vi "Deposit Amount.vi"(10 "User Input":string, 11 "Module Data in":T1) -> (2 "Deposit Complete Message":string, 3 "Module Data out":T1)   [LabVIEW 2016]
uses:
  <vilib>/Utility/file.llb/Write Delimited Spreadsheet (string).vi
  Controls/UI Controls.ctl
  Controls/ATM Messages.ctl
  Controls/Transaction Status.ctl
  Controls/User Input Data.ctl
  Controls/Module Data.ctl
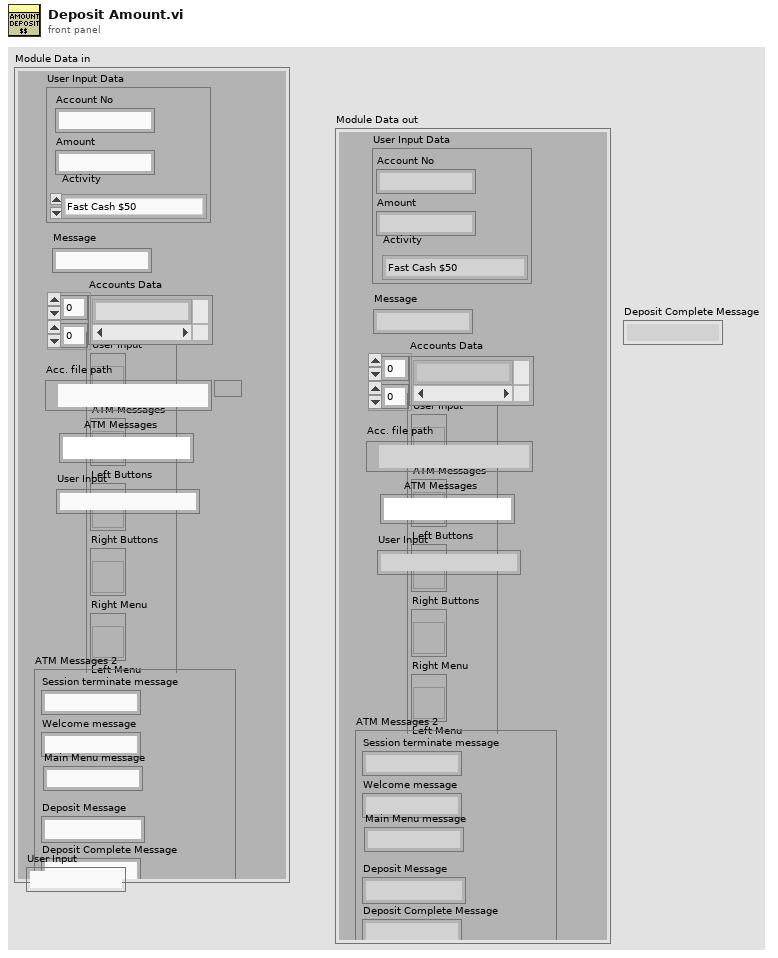
[diagram p1: front panel]
types:
  T1 = typedef "Module Data.ctl" = cluster{"UI Controls":T2, "ATM Messages 2":T3, "User Input":string, "ATM Messages":string, "Acc. file path":path, "Accounts Data":string[][], "User Input Data":T4, "Message":string}
  T2 = typedef "UI Controls.ctl" = cluster{"ATM Messages":refnum<vi>, "User Input":refnum<vi>, "Right Buttons":refnum<vi>, "Right Menu":refnum<vi>, "Left Buttons":refnum<vi>, "Left Menu":refnum<vi>, "Card Simulator":refnum<vi>, "Enter":refnum<vi>}
  T3 = typedef "ATM Messages.ctl" = cluster{"Session terminate message":string, "Welcome message":string, "Deposit Message":string, "Deposit Complete Message":string, "Withdrawal Message":string, "Withdrawal Complete Message":string, "Balance Inquiry Message":string, "Account verification failed message":string, "Withdrawal failed message":string, "Card Inserted":string, "Main Menu message":string}
  T4 = typedef "User Input Data.ctl" = cluster{"Account No":string, "Amount":string, "Activity":T5}
  T5 = typedef "Transaction Status.ctl" = enum16{"Fast Cash $50", "Withdrawal?", "Deposit?", "Account Number?"}
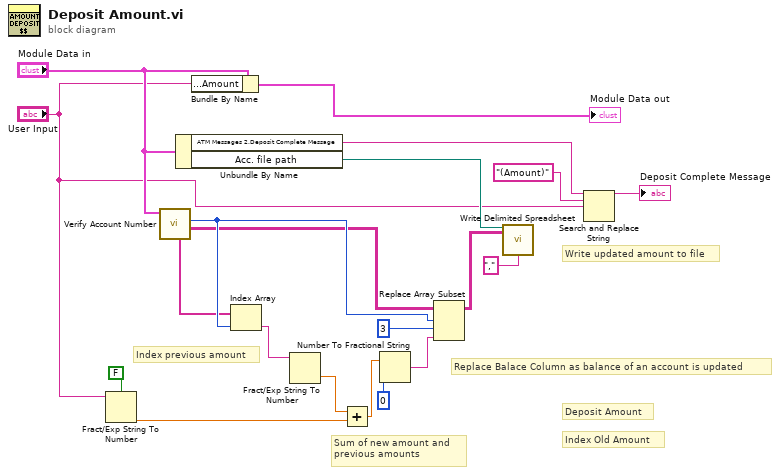
[diagram p0: block diagram]
diagram:
  # "Write updated amount to file"
  # "Sum of new amount and\nprevious amounts"
  # "Index previous amount"
  # "Replace Balace Column as balance of an account is updated"
  # "Index Old Amount"
  # "Deposit Amount"
  n1 = Fract/Exp String To Number(use system decimal point (T)=FALSE, string="User Input") -> (number=w16:dbl)  [unwired: 2 in, 1 out]
  n2 = call "Verify Account Number.vi"("Module Data"="Module Data in") -> ("Accounts all data"=w8:string[][], "Index account no."=w13:i32, "Balances Column"=w7:string[])  [unwired: 6 in, 2 out]
  n3 = Unbundle By Name("Module Data in") -> ("ATM Messages 2.Deposit Complete Message"=w3:string, "Acc. file path"=w9:path)
  n4 = Bundle By Name(cluster="Module Data in", "User Input Data.Amount"="User Input") -> (→"Module Data out":T1)
  n5 = Index Array(array=w7, index=w13) -> (element=w17:string)
  n6 = Fract/Exp String To Number(string=w17) -> (number=w18:dbl)  [unwired: 3 in, 1 out]
  n7 = Add(x=w18, y=w16) -> (x+y=w19:dbl)
  n8 = Number To Fractional String(number=w19, precision (6)=i16 0) -> (F-format string=w5:string)  [unwired: 2 in]
  n9 = Replace Array Subset(array=w8, new element=w5, index (row)=w13, index (col)=3 ("disabled index (col)")) -> (w12:string[][])
  n10 = call-poly <vilib>:"Write Delimited Spreadsheet.vi"("file path (dialog if empty)"=w9, "2D data"=w12, "delimiter (\\t)"="," ("delimiter (\\t)")) -> ()  [unwired: 11 in, 2 out]
  n11 = Search and Replace String(input string=w3, search string="(Amount)" ("search string/char (-)"), replace string="User Input") -> (result string=→"Deposit Complete Message":string)  [unwired: 5 in, 3 out]
